vi "sub_trigger-check.vi"(8 "error in (no error)":errorcluster caption="에러 입력(에러 없음)", 11 "wf history":waveform(dbl)[][](array[waveform])) -> (0 "error out":errorcluster caption="에러 출력", 3 "stop triiger":bool)   [LabVIEW 2013]
uses:
  Global.vi
panel:
  out "main":bool
  out "sub":bool
  out "크기":i32[](array[numeric])
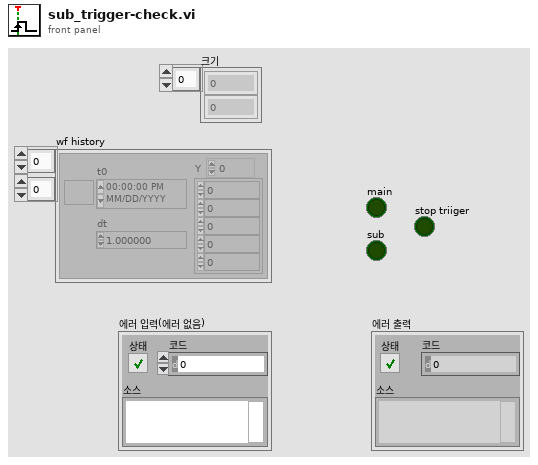
[diagram p1: front panel]
types:
  T1 = typedef "config_ctl.ctl" = cluster{"Trigger minlevel":dbl, "Lower Cut-Off":dbl, "Vacuum Trigger level":dbl, "state settings":cluster{"method":enum32{"histogram", "peak", "auto select"}, "histogram size":i32, "histogram method":enum16{"mode"}, "reserved":dbl}, "SPA-300 Setting":cluster{"Bonding force (g)":dbl, "Bonding time (ms)":dbl, "Pickup force (g)":dbl, "Pickup time (ms)":dbl, "Speed":enum16{"Slow", "Fast"}}}
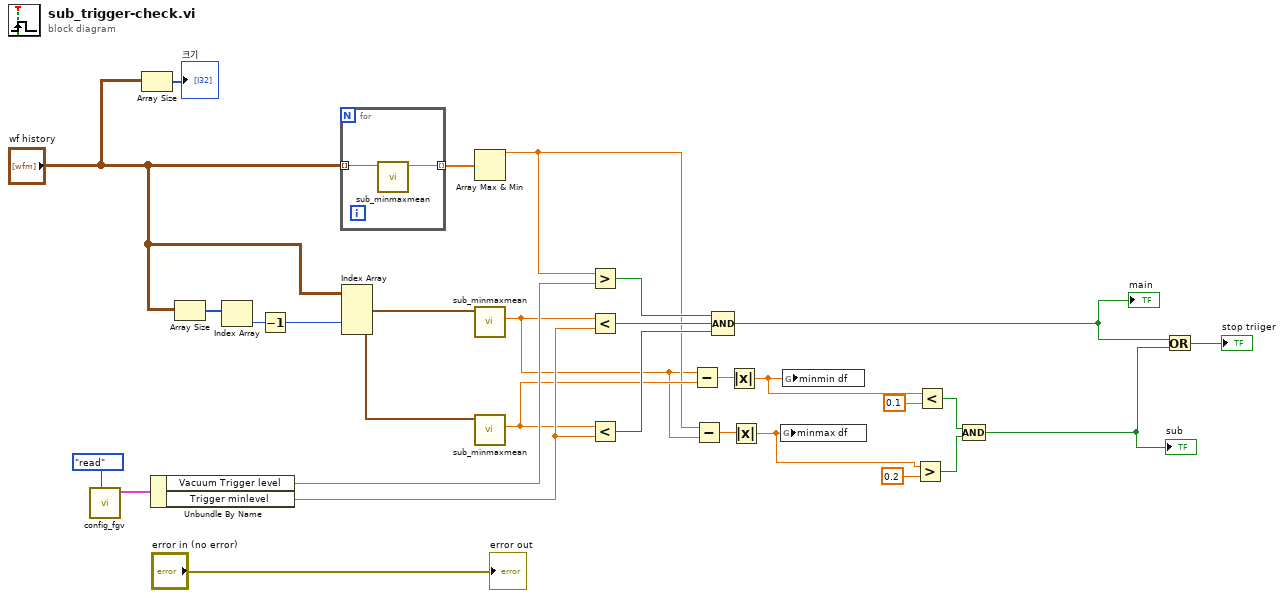
[diagram p0: block diagram]
diagram:
  n1 = call "config_fgv.vi"("cmd"=enum16{"write", "read", "ini"}."read") -> ("Config out"=w22:T1)  [unwired: 9 in, 1 out]
  n2 = Array Size(array="wf history") -> (size(s)=→"크기":i32[])
  n3 = Unbundle By Name(w22) -> ("Vacuum Trigger level"=w20:dbl, "Trigger minlevel"=w21:dbl)
  n4 = Array Size(array="wf history") -> (size(s)=w30:i32[])
  n5 = Index Array(array=w30) -> (element=w29:i32)  [unwired: 1 in]
  n6 = Decrement(x=w29) -> (x-1=w28:i32)
  n7 = for {
    tunnel: "wf history" -> [w31] mode=indexing
    tunnel: [w32] -> w27 mode=indexing
    n8 = call "sub_minmaxmean.vi"("History Data"=w31) -> ("mean"=w32:dbl)  [unwired: 8 in, 2 out]
  }
  n9 = Index Array(array="wf history", index (row) #2=w28) -> (element #1=w18:waveform(dbl)[], element #2=w19:waveform(dbl)[])  [unwired: 3 in]
  n10 = Array Max & Min(array=w27) -> (max value=w13:dbl)  [unwired: 3 out]
  n11 = call "sub_minmaxmean.vi"("History Data"=w18) -> ("max"=w12:dbl)  [unwired: 8 in, 2 out]
  n12 = call "sub_minmaxmean.vi"("History Data"=w19) -> ("max"=w16:dbl)  [unwired: 8 in, 2 out]
  n13 = Greater?(x=w13, y=w20) -> (0:w26:bool)
  n14 = Less?(x=w12, y=w21) -> (x < y?=w25:bool)
  n15 = Less?(x=w16, y=w21) -> (x < y?=w24:bool)
  n16 = Subtract(x=w12, y=w16) -> (x-y=w15:dbl)
  n17 = Subtract(x=w13, y=w12) -> (x-y=w14:dbl)
  n18 = Compound Arithmetic op=AND(w26, w25, w24) -> (w2:bool)
  "main" <- w2
  n19 = Absolute Value(x=w15) -> (abs(x)=w9:dbl)
  n20 = Absolute Value(x=w14) -> (abs(x)=w6:dbl)
  n21 = global write "Global.vi" "minmax df"(w6) -> ()
  n22 = global write "Global.vi" "minmin df"(w9) -> ()
  n23 = Greater?(x=w6, y=0.2) -> (0:w5:bool)
  n24 = Less?(x=w9, y=0.1) -> (x < y?=w4:bool)
  n25 = Compound Arithmetic op=AND(w4, w5) -> (w3:bool)
  "sub" <- w3
  n26 = Or(x=w2, y=w3) -> (x .or. y?=→"stop triiger":bool)
  "error out" <- "error in (no error)"
